vi "_FPGA Toggle LED.vi"(5 "error in (no error)":errorcluster, 6 "OFF State (P)":T1=enum."Off P", 7 "ON State (P)":T1=enum."Solid P") -> (0 "error out":errorcluster)   [LabVIEW 2015]
uses:
  Type/_LED States.ctl
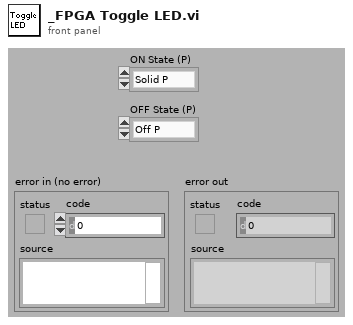
[diagram p1: front panel]
types:
  T1 = typedef "_LED States.ctl" = enum8{"Idle", "Solid B", "Solid R", "Solid P", "Off B", "Off R", "Off P", "Off BRP", "Off RP", "Flash R&P", "Flash P"}
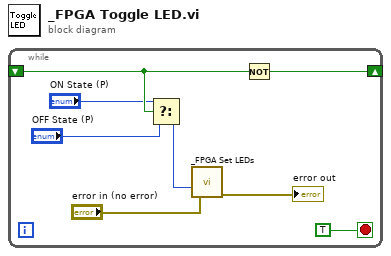
[diagram p0: block diagram]
diagram:
  n1 = while {
    shift-right: [w5] -> _
    shift-left: _ -> [w4]
    stop <- TRUE stop-if-true
    n2 = Select(t="ON State (P)", s=w4, f="OFF State (P)") -> (s? t:f=w1:T1)
    n3 = call "_FPGA Set LEDs.vi"("error in (no error)"="error in (no error)", "LED Command"=w1) -> ("error out"=→"error out":errorcluster)  [unwired: 2 in, 3 out]
    n4 = Not(x=w4) -> (.not. x?=w5:bool)
  }
